vi "Adressen schreiben.vi"(8 "error in (no error)":errorcluster caption="Fehler (Eingang, kein Fehler)", 10 "Adressen":T1, 11 "Steuerung PNS (Eingang)":refnum<class "Steuerung PNS.lvclass">) -> (0 "error out":errorcluster caption="Fehler (Ausgang)", 3 "Steuerung PNS (Ausgang)":refnum<class "Steuerung PNS.lvclass">)   [LabVIEW 2020, in "Steuerung PNS.lvclass"]
uses:
  Steuerung PNS.lvclass
  Adresse.ctl
  Steuerung PNS.lvclass/Steuerung PNS.ctl
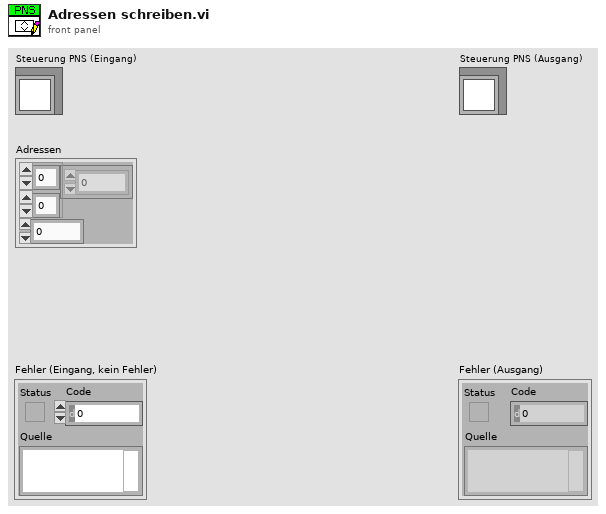
[diagram p1: front panel]
types:
  T1 = typedef "Steuerung PNS.lvclass/Adresse.ctl" = cluster{i32[][], i32}
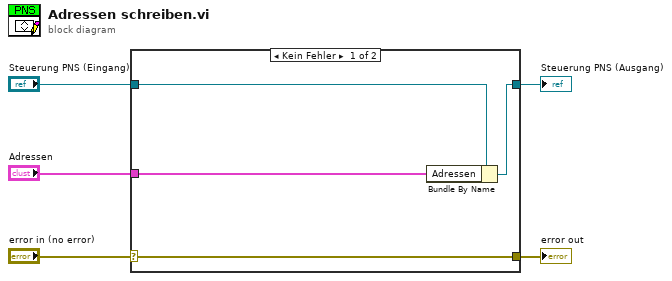
[diagram p0: block diagram]
diagram:
  n1 = case shown="Kein Fehler" "error in (no error)" {
    selector: "error in (no error)" -> [w9 w10]
    tunnel: [w9 w10] -> w4
    tunnel: [w7 w11] -> w2
    tunnel: "Steuerung PNS (Eingang)" -> [w8 w11]
    tunnel: "Adressen" -> [w6 _]
    frame No Error {
      n2 = Bundle By Name(cluster=w8, "Adressen"=w6) -> (w7:refnum<class "Steuerung PNS.lvclass">)
    }
    frame Error {
    }
  }
  "error out" <- w4
  "Steuerung PNS (Ausgang)" <- w2
